vi "SubVI_buttons_teleop.vi"(11 "Buttons":bool[](array[boolean])) -> ()   [LabVIEW 2017]
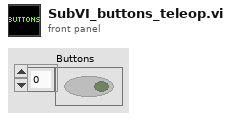
[diagram p1: front panel]
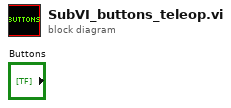
[diagram p0: block diagram]
diagram:
